vi "Read_calibration_files.vi"() -> ()   [LabVIEW 2022 SP3]
uses:
  Controls/Pressure_Units.ctl
  Controls/Post_Process.ctl
  Controls/Instrument_Array.ctl
  Controls/Inst_type.ctl
  Globals/Meas_global.vi
  Globals/Trav_pos_global.vi
  Acquisition/PWA/PWAtasksGLOBAL.vi
panel:
  in  "Pressure Units":T1
  # "This Program Read data in from the calibration files"
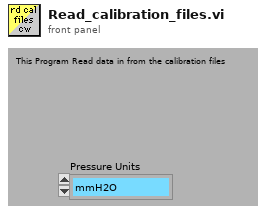
[diagram p1: front panel]
types:
  T1 = typedef "Pressure_Units.ctl" = enum16{"mmH2O", "mmHg", "Pa (N/m^2)", "mbar", "bar"}
  T2 = typedef "Analysis_info_cluster.ctl" = cluster{"Colour":u32, "Inst type":T3, "Inst name":string, "Symbol":string, "Code name":string, "Extra Info":string, "Inst Array":T4, "Extra Titles":string[], "Extra Values":string[], "U":dbl, "u^2":dbl, "u^3":dbl, "u^4":dbl, "Skew_u":dbl, "Kurt_u":dbl, "Sd Error in Mean":dbl, "% u'/U":dbl, "X":dbl, "Y":dbl, "Z":dbl, "Timescale integral Estimate":dbl, "Sd Error in Variance":dbl, "Calib File":path, "Calib Constants":dbl[], "Output Position":bool, "Stats":enum16{"None", "Basic", "Full"}, "Av Sampling Rate":dbl, "Av No of Samples":dbl, "Total Meas Time (s)":dbl, "ADAM Ch Name":string, "Max value":dbl, "Min value":dbl, "Req Sample Rate Hz":dbl, "Sync Delay Time (s)":dbl, "Ch No":i16, "Device":string, "Use Latest Calib":bool, "Port":string, "Metadata Ch Names":string[], "Metadata Ch Values":string[], "Label":string, "chState":T5, "Point Drift":dbl}
  T3 = typedef "Inst_type.ctl" = enum16{"Raw voltage", "Raw with zero offsetting", "Propeller anemometer", "Pressure Transducer", "Pitot-static tube", "Hot wire", "Cross wire 1", "Cross wire 2", "Generic Linear", "Generic Polynomial", "Generic BackPoly", "Fast FID", "Thermocouple", "Cold wire", "Pulsed Wire", "LDA Vel", "LDA Tran time", "LDA Arr time", "Microphone"}
  T4 = typedef "Instrument_Array.ctl" = enum16{"PWA", "LDA", "Analogue"}
  T5 = typedef "channelState.ctl" = enum32{"No Selection", "Solo", "Mute"}
  T6 = typedef "PWA_Data.ctl" = enum16{"No PWA Data", "One Ch PWA"}
  T7 = typedef "Post_Process.ctl" = enum16{"Take New Data", "Post Process Raw Data File"}
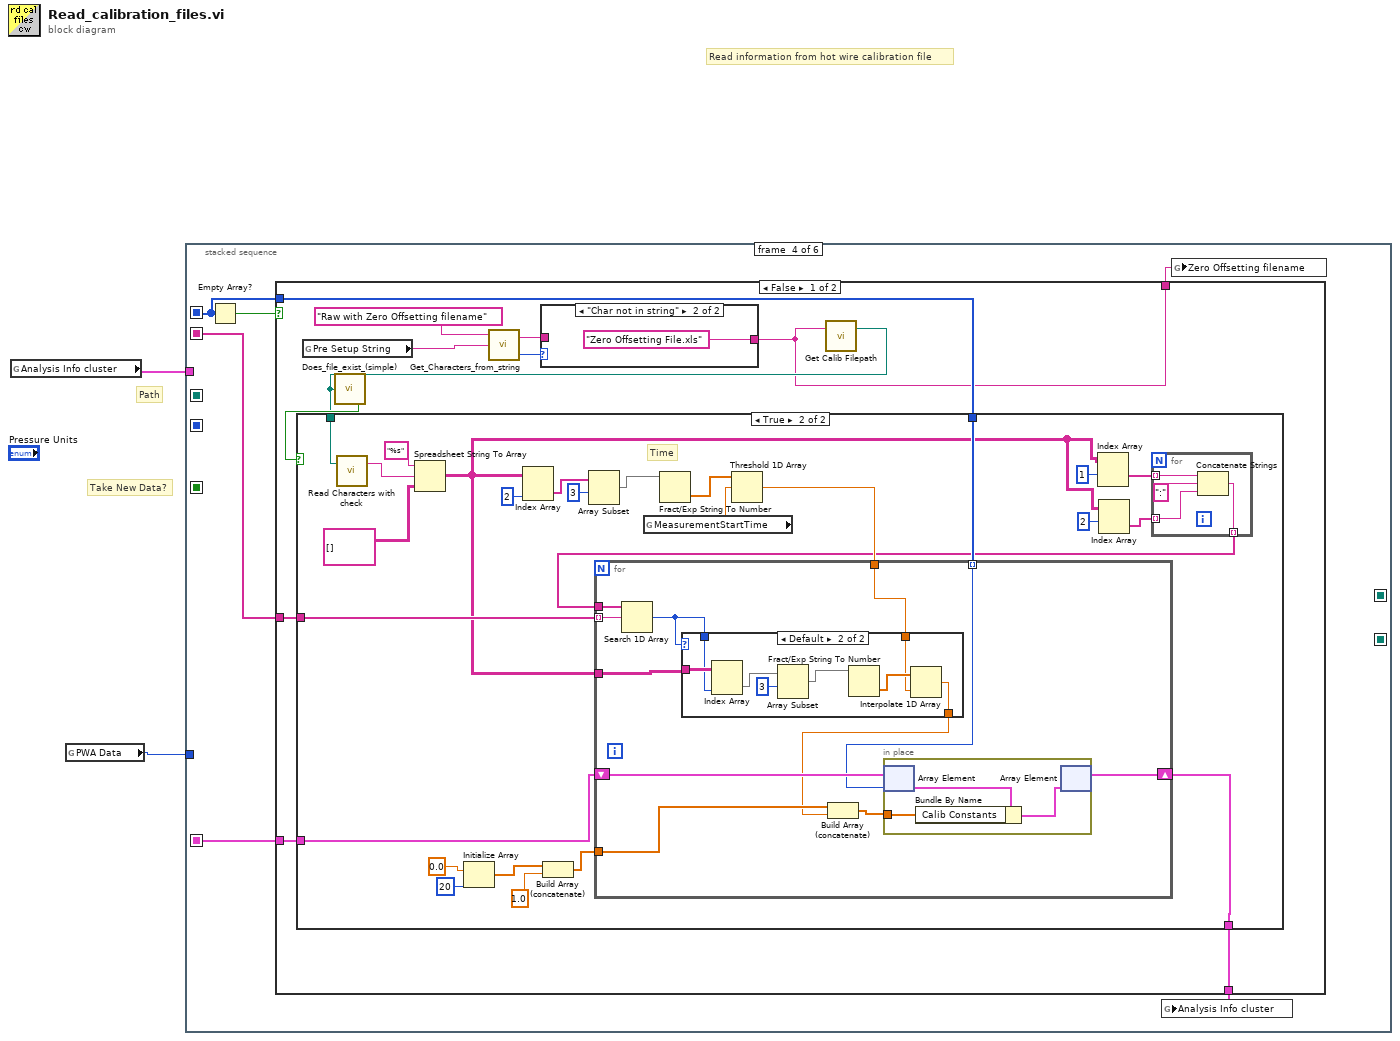
[diagram p0: block diagram]
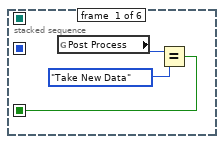
[diagram p2: hidden frame]
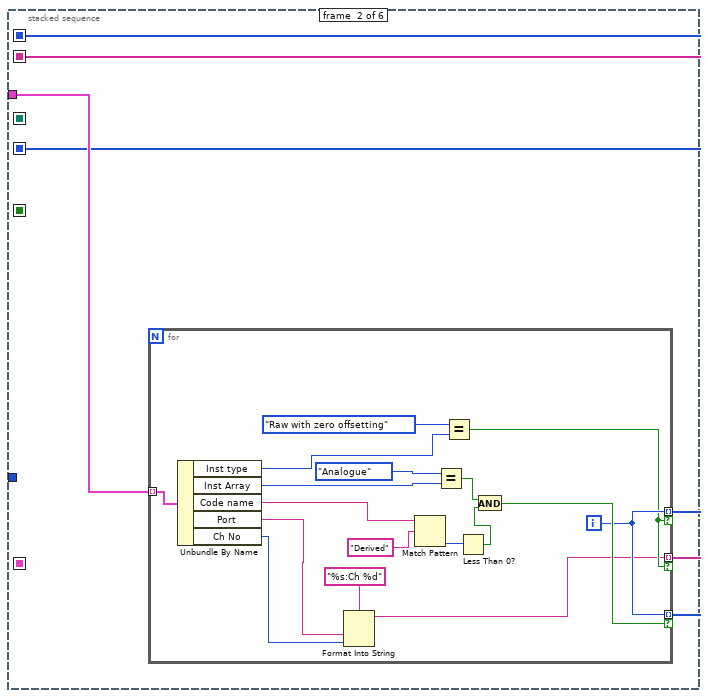
[diagram p3: hidden frame]
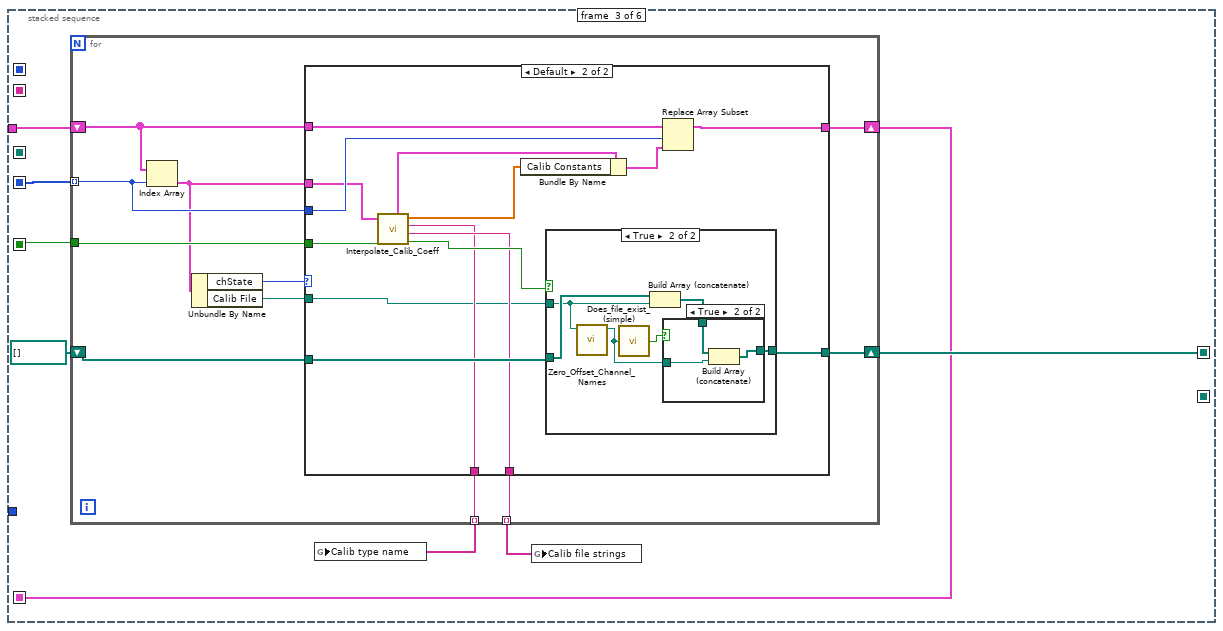
[diagram p4: hidden frame]
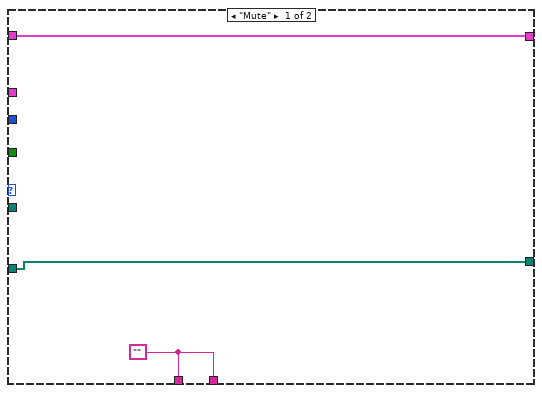
[diagram p5: hidden frame]
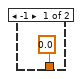
[diagram p10: hidden frame]
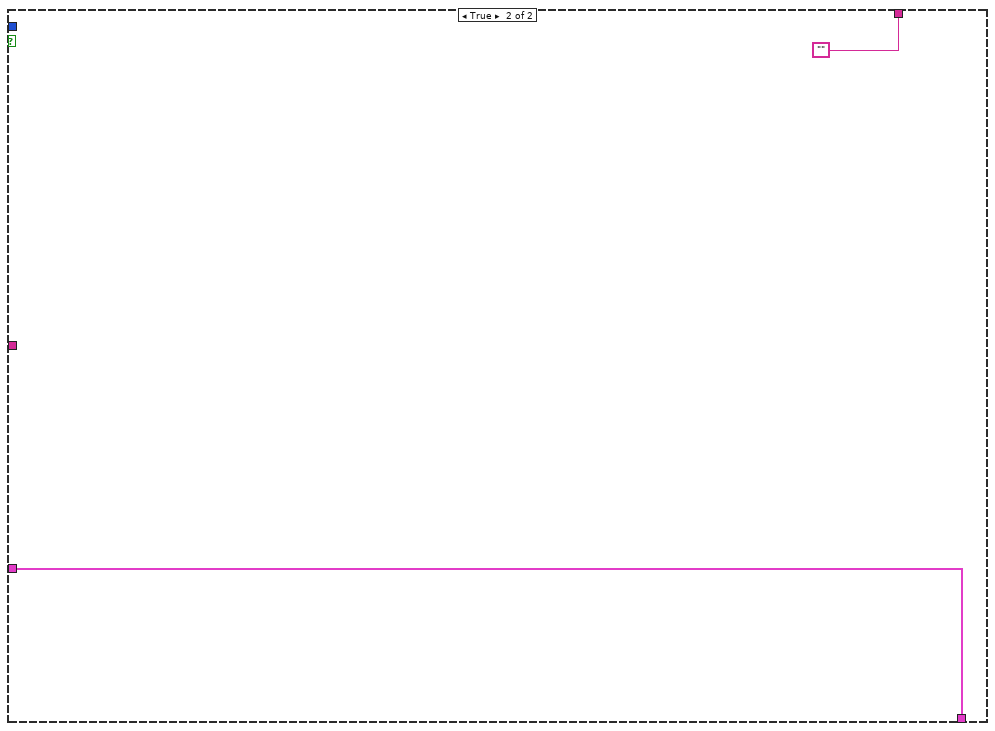
[diagram p11: hidden frame]
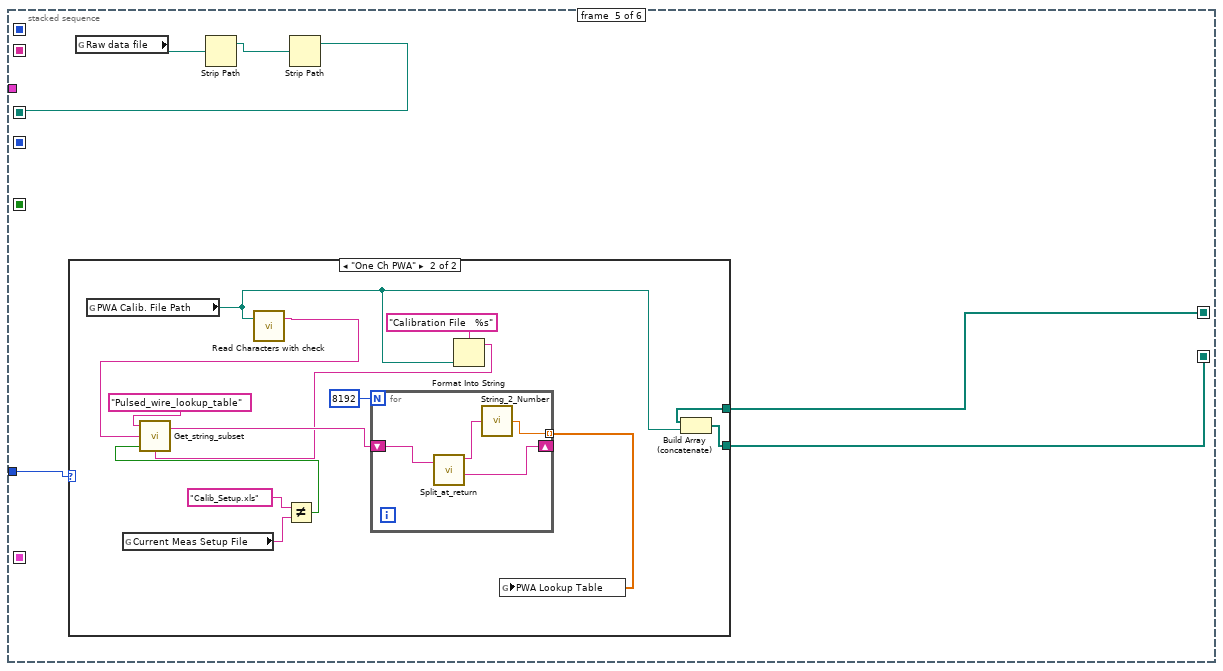
[diagram p12: hidden frame]
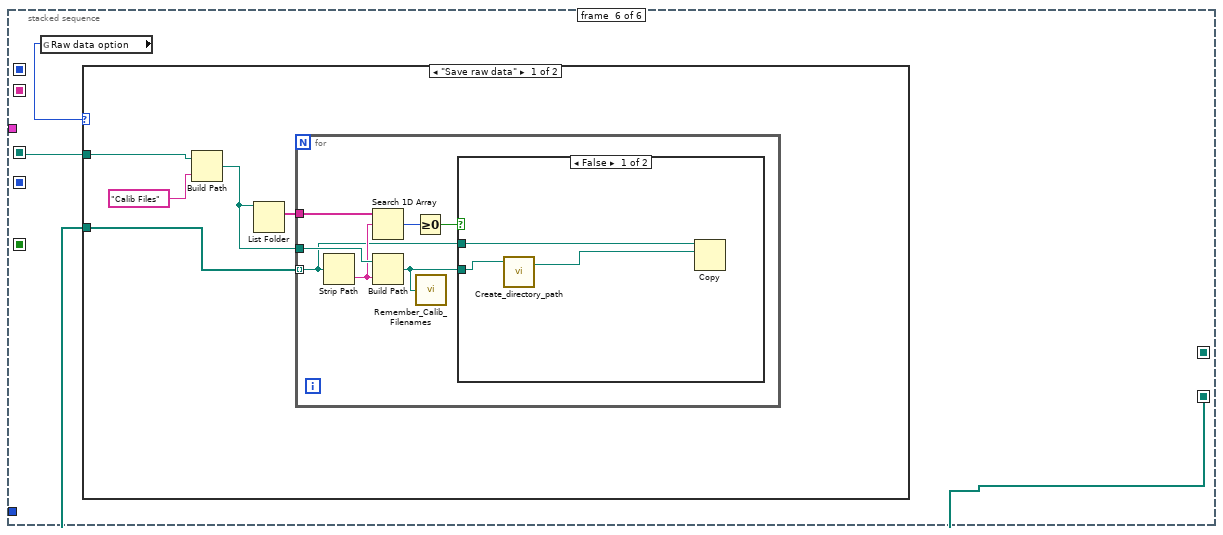
[diagram p14: hidden frame]
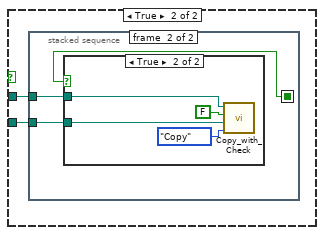
[diagram p15: hidden frame]
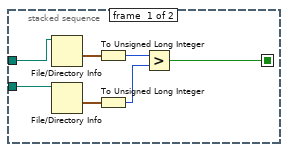
[diagram p16: hidden frame]
diagram:
  # "Take New Data?"
  # "Path"
  # "Read information from hot wire calibration file"
  n1 = global read "Meas_global.vi" "Analysis Info cluster"() -> (w1:T2[])
  n2 = global read "Meas_global.vi" "PWA Data"() -> (w2:T6)
  n3 = stacked-sequence {
    seq-local: [_ _ w34 _ _ _] -> [_ _ _ _ w151 _]
    seq-local: [_ _ _ _ w149 _] -> [_ _ _ _ _ w174]
    seq-local: [w3 _ _ _ _ _] -> [_ _ w32 _ _ _]
    seq-local: [_ _ _ _ w152 _] -> [_ _ _ _ _ w173]
    seq-local: [_ w8 _ _ _ _] -> [_ _ w28 _ _ _]
    seq-local: [_ _ w27 _ _ _] -> [_ _ _ w79 _ _]
    seq-local: [_ w7 _ _ _ _] -> [_ _ _ w77 _ _]
    seq-local: [_ w6 _ _ _ _] -> [_ _ _ w75 _ _]
    tunnel: w2 -> [_ _ _ _ w153 _]
    tunnel: w1 -> [_ w9 w29 _ _ _]
    frame #0 {
      n4 = global read "Meas_global.vi" "Post Process"() -> (w4:T7)
      n5 = Equal?(x=w4, y=Post_Process."Take New Data" ("Post Process")) -> (x = y?=w3:bool)
    }
    frame #1 {
      n6 = for {
        tunnel: w9 -> [w20] mode=indexing
        tunnel: [w16] -> w8 mode=indexing if=w17
        tunnel: [w16] -> w7 mode=indexing if=w14
        tunnel: [w10] -> w6 mode=indexing if=w14
        i -> [w16]
        n7 = Unbundle By Name(w20) -> ("Inst type"=w19:T3, "Inst Array"=w26:T4, "Code name"=w15:string, "Port"=w12:string, "Ch No"=w11:i16)
        n8 = Format Into String(format string="%s:Ch %d", w12, w11) -> (resulting string=w10:string)  [unwired: 2 in, 1 out]
        n9 = Match Pattern(string=w15, regular expression="Derived") -> (offset past match=w23:i32)  [unwired: 4 out]
        n10 = Equal?(x=Instrument_Array."Analogue" ("Inst Array"), y=w26) -> (x = y?=w21:bool)
        n11 = Equal?(x=Inst_type."Raw with zero offsetting", y=w19) -> (x = y?=w14:bool)
        n12 = Less Than 0?(x=w23) -> (x < 0?=w22:bool)
        n13 = And(x=w21, y=w22) -> (x .and. y?=w17:bool)
      }
    }
    frame #2 {
      n14 = for {
        shift-right: [w44] -> w34
        shift-left: path[] [] -> [w45]
        tunnel: w32 -> [w43]
        tunnel: [w42] -> w31 mode=indexing
        tunnel: [w41] -> w30 mode=indexing
        shift-right: [w38] -> w27
        shift-left: w29 -> [w40]
        tunnel: w28 -> [w39] mode=indexing
        n15 = Index Array(array=w40, index=w39) -> (element=w37:T2)
        n16 = Unbundle By Name(w37) -> ("chState"=w35:T5, "Calib File"=w36:path)
        n17 = case shown="Default" w35 {
          tunnel: w45 -> [w47 w62]
          tunnel: [w47 w61] -> w44
          tunnel: w43 -> [_ w60]
          tunnel: [w46 w58] -> w42
          tunnel: [w46 w57] -> w41
          tunnel: w40 -> [w48 w56]
          tunnel: w39 -> [_ w55]
          tunnel: [w48 w54] -> w38
          tunnel: w37 -> [_ w50]
          tunnel: w36 -> [_ w49]
          frame "Mute" {
            w46 = ""
          }
          frame Default {
            n18 = call "Interpolate_Calib_Coeff.vi"("Analysis Info cluster"=w50, "Take New Data?"=w60) -> ("Calib Coeff"=w51:dbl[], "Calib Type Name"=w57:string, "Calib file string"=w58:string, "Read file"=w59:bool, "Analysis Info cluster  Out"=w53:T2)  [unwired: 1 in]
            n19 = Bundle By Name(cluster=w53, "Calib Constants"=w51) -> (w52:T2)
            n20 = case shown="True" w59 {
              tunnel: w62 -> [w63 w69]
              tunnel: [w63 w64] -> w61
              tunnel: w49 -> [_ w68]
              frame False {
              }
              frame True {
                n21 = call "Zero_Offset_Channel_Names.vi"("Calib Filename"=w68) -> ("Zero Filename"=w65:path)  [unwired: 3 in, 3 out]
                n22 = call "Does_file_exist_(simple).vi"("Pathname"=w65) -> ("exists?"=w67:bool)
                n23 = Build Array (concatenate)(w69, w68) -> (w66:path[])
                n24 = case shown="True" w67 {
                  tunnel: w66 -> [w70 w73]
                  tunnel: w65 -> [_ w72]
                  tunnel: [w70 w71] -> w64
                  frame False {
                  }
                  frame True {
                    n25 = Build Array (concatenate)(w73, w72) -> (w71:path[])
                  }
                }
              }
            }
            n26 = Replace Array Subset(array=w56, new element=w52, index=w55) -> (w54:T2[])
          }
        }
      }
      n27 = global write "Meas_global.vi" "Calib type name"(w30) -> ()
      n28 = global write "Meas_global.vi" "Calib file strings"(w31) -> ()
    }
    frame #3 {
      n29 = Empty Array?(array=w77) -> (empty?=w78:bool)
      n30 = case shown="False" w78 {
        tunnel: w79 -> [w88 w148]
        tunnel: w77 -> [w87 _]
        tunnel: [w86 w148] -> w76
        tunnel: w75 -> [w83 _]
        tunnel: [w81 ""] -> w74
        frame False {
          n31 = global read "Meas_global.vi" "Pre Setup String"() -> (w84:string)
          n32 = call "Get_Characters_from_string.vi"("Input string"=w84, "Variable name"="Raw with Zero Offsetting filename" ("Label for characters")) -> ("Status"=w82:enum16{"Char in string", "Char not in string"}, "Value"=w80:string)  [unwired: 1 in]
          n33 = case shown="\"Char not in string\"" w82 {
            tunnel: [w91 "Zero Offsetting File.xls" ("Filename String")] -> w81
            tunnel: w80 -> [w91 _]
            frame "Char in string" {
            }
            frame "Char not in string" {
            }
          }
          n34 = call "Get Calib Filepath.vi"("Filename String"=w81) -> ("Filename Out"=w89:path)  [unwired: 2 in]
          n35 = call "Does_file_exist_(simple).vi"("Pathname"=w89) -> ("exists?"=w90:bool)
          n36 = case shown="True" w90 {
            tunnel: w89 -> [_ w101]
            tunnel: w88 -> [w93 w108]
            tunnel: w87 -> [_ w106]
            tunnel: [w93 w107] -> w86
            tunnel: w83 -> [_ w105]
            frame False {
            }
            frame True {
              # "Time"
              n37 = call "Read Characters with check.vi"("file (use dialog)"=w101) -> ("Read String"=w100:string)  [unwired: 1 in, 1 out]
              n38 = Spreadsheet String To Array(format string="%s", spreadsheet string=w100, array type (2D Dbl)=string[][] []) -> (array=w94:string[][])  [unwired: 1 in]
              n39 = Initialize Array(0.0, 20 ("dimension size")) -> (w103:dbl[])
              n40 = Index Array(array=w94, index (col)=2 ("disabled index (col)")) -> (element=w115:string[])  [unwired: 1 in]
              n41 = Build Array (concatenate)(w103, 1.0) -> (w104:dbl[])
              n42 = Array Subset(array=w115, index=3) -> (w117:string[])  [unwired: 1 in]
              n43 = global read "Meas_global.vi" "MeasurementStartTime"() -> (w112:dbl)
              n44 = Fract/Exp String To Number(string=w117) -> (number=w113:dbl[])  [unwired: 3 in, 1 out]
              n45 = Threshold 1D Array(2:w112, 3:w113) -> (0:w111:dbl)  [unwired: 1 in]
              n46 = Index Array(array=w94, index (row)=1) -> (element=w97:string[])  [unwired: 1 in]
              n47 = Index Array(array=w94, index (row)=2) -> (element=w96:string[])  [unwired: 1 in]
              n48 = for {
                tunnel: w97 -> [w123] mode=indexing
                tunnel: w96 -> [w122] mode=indexing
                tunnel: [w120] -> w95 mode=indexing
                n49 = Concatenate Strings(w123, ":" ("string"), w122) -> (w120:string)
              }
              n50 = for {
                tunnel: w94 -> [w134]
                tunnel: w111 -> [w133]
                shift-right: [w131] -> w107
                shift-left: w108 -> [w132]
                tunnel: w104 -> [w130]
                tunnel: w106 -> [w127] mode=indexing
                tunnel: w95 -> [w126]
                tunnel: w105 -> [w125] mode=indexing
                n51 = Search 1D Array(1D array=w126, element=w125) -> (index of element=w124:i32)  [unwired: 1 out]
                n52 = case shown="Default" w124 {
                  tunnel: w134 -> [_ w140]
                  tunnel: w133 -> [_ w138]
                  tunnel: [0.0 w137] -> w129
                  tunnel: w124 -> [_ w136]
                  frame -1 {
                  }
                  frame Default {
                    n53 = Index Array(array=w140, index (col)=w136) -> (element=w143:string[])  [unwired: 1 in]
                    n54 = Array Subset(array=w143, index=3) -> (w141:string[])  [unwired: 1 in]
                    n55 = Fract/Exp String To Number(string=w141) -> (number=w139:dbl[])  [unwired: 3 in, 1 out]
                    n56 = Interpolate 1D Array(1:w138, 2:w139) -> (0:w137:dbl)
                  }
                }
                n57 = Build Array (concatenate)(w130, w129) -> (w128:dbl[])
                n58 = in-place {
                  in-place-border: w128 -> [w144]
                  n59 = in-place-array #1(w132, w127) -> (w146:T2)
                  n60 = Bundle By Name(cluster=w146, "Calib Constants"=w144) -> (w145:T2)
                  n61 = in-place-array #1(w145) -> (w131:T2[])  [unwired: 1 out]
                }
              }
            }
          }
        }
        frame True {
        }
      }
      n62 = global write "Meas_global.vi" "Analysis Info cluster"(w76) -> ()
      n63 = global write "Meas_global.vi" "Zero Offsetting filename"(w74) -> ()
    }
    frame #4 {
      n64 = case shown="\"One Ch PWA\"" w153 {
        tunnel: [w155 w160] -> w152
        tunnel: w151 -> [w155 w161]
        frame "No PWA Data" {
        }
        frame "One Ch PWA" {
          n65 = global read "PWAtasksGLOBAL.vi" "PWA Calib. File Path"() -> (w157:path)
          n66 = global read "Trav_pos_global.vi" "Current Meas Setup File"() -> (w167:string)
          n67 = call "Read Characters with check.vi"("file (use dialog)"=w157) -> ("Read String"=w156:string)  [unwired: 1 in, 1 out]
          n68 = Not Equal?(x="Calib_Setup.xls", y=w167) -> (x != y?=w168:bool)
          n69 = Format Into String(format string="Calibration File   %s", w157) -> (resulting string=w158:string)  [unwired: 2 in, 1 out]
          n70 = call "Get_string_subset.vi"("String Name"=w158, "Show Dialog?"=w168, "String to split"=w156, "File Label"="Pulsed_wire_lookup_table") -> ("Output string"=w163:string)  [unwired: 1 out]
          n71 = for {
            N: 8192 -> [_]
            shift-right: [w171] -> _
            shift-left: w163 -> [w172]
            tunnel: [w169] -> w164 mode=indexing
            n72 = call "Split_at_return.vi"("String"=w172) -> ("before substring"=w170:string, "after substring"=w171:string)  [unwired: 1 in, 2 out]
            n73 = call "String_2_Number.vi"("Value"=w170) -> ("Numeric"=w169:dbl)
          }
          n74 = global write "PWAtasksGLOBAL.vi" "PWA Lookup Table"(w164) -> ()
          n75 = Build Array (concatenate)(w161, w157) -> (w160:path[])
        }
      }
      n76 = global read "Meas_global.vi" "Raw data file"() -> (w154:path)
      n77 = Strip Path(path=w154) -> (stripped path=w150:path)  [unwired: 1 out]
      n78 = Strip Path(path=w150) -> (stripped path=w149:path)  [unwired: 1 out]
    }
    frame #5 {
      n79 = global read "Meas_global.vi" "Raw data option"() -> (w175:enum16{"Save raw data", "Raw data not saved"})
      n80 = case shown="\"Save raw data\"" w175 {
        tunnel: w173 -> [w180 _]
        tunnel: w174 -> [w178 _]
        frame "Save raw data" {
          n81 = Build Path(base path=w178, name or relative path="Calib Files" ("format string")) -> (appended path=w176:path)
          n82 = List Folder(path=w176) -> (filenames=w179:string[])  [unwired: 1 in, 5 out]
          n83 = for {
            tunnel: w180 -> [w181] mode=indexing
            tunnel: w176 -> [w184]
            tunnel: w179 -> [w187]
            n84 = Strip Path(path=w181) -> (name=w183:string)  [unwired: 1 out]
            n85 = Search 1D Array(1D array=w187, element=w183) -> (index of element=w186:i32)  [unwired: 1 out]
            n86 = Build Path(base path=w184, name or relative path=w183) -> (appended path=w182:path)
            n87 = Greater Or Equal To 0?(x=w186) -> (x >= 0?=w185:bool)
            n88 = call "Remember_Calib_Filenames.vi"("Filename to Remember"=w182) -> ()  [unwired: 1 out]
            n89 = case shown="False" w185 {
              tunnel: w182 -> [w189 w191]
              tunnel: w181 -> [w190 w192]
              frame False {
                n90 = call "Create_directory_path.vi"("Path name"=w189) -> ("Path name Out"=w188:path)  [unwired: 2 in, 1 out]
                n91 = Copy(10:w188, 11:w190) -> ()  [unwired: 1 in, 5 out]
              }
              frame True {
                n92 = stacked-sequence {
                  seq-local: [w195 _] -> [_ w202]
                  tunnel: w192 -> [w199 w200]
                  tunnel: w191 -> [w198 w201]
                  frame #0 {
                    n93 = File/Directory Info(path=w199) -> (last mod=w193:timestamp)  [unwired: 1 in, 6 out]
                    n94 = File/Directory Info(path=w198) -> (last mod=w194:timestamp)  [unwired: 1 in, 6 out]
                    n95 = To Unsigned Long Integer(number=w193) -> (unsigned 32bit integer=w197:u32)
                    n96 = To Unsigned Long Integer(number=w194) -> (unsigned 32bit integer=w196:u32)
                    n97 = Greater?(x=w197, y=w196) -> (0:w195:bool)
                  }
                  frame #1 {
                    n98 = case shown="True" w202 {
                      tunnel: w201 -> [_ w203]
                      tunnel: w200 -> [_ w206]
                      frame False {
                      }
                      frame True {
                        n99 = call "Copy_with_Check.vi"("Mode"=enum16{"Move", "Copy"}."Copy", "Target Path"=w203, "Variable Target?"=FALSE, "Source Path"=w206) -> ()  [unwired: 1 out]
                      }
                    }
                  }
                }
              }
            }
          }
        }
        frame "Raw data not saved" {
        }
      }
    }
  }
